vi "Actualizar Parametros.vi"(8 "error in (no error)":errorcluster, 10 "Parametros de la señal":T1, 11 "Generador de Señales in":refnum<class "Generador de Señales.lvclass">) -> (0 "error out":errorcluster, 3 "Generador de Señales out":refnum<class "Generador de Señales.lvclass">)   [LabVIEW 2020, in "Generador de Señales.lvlib" / "Generador de Señales.lvclass"]
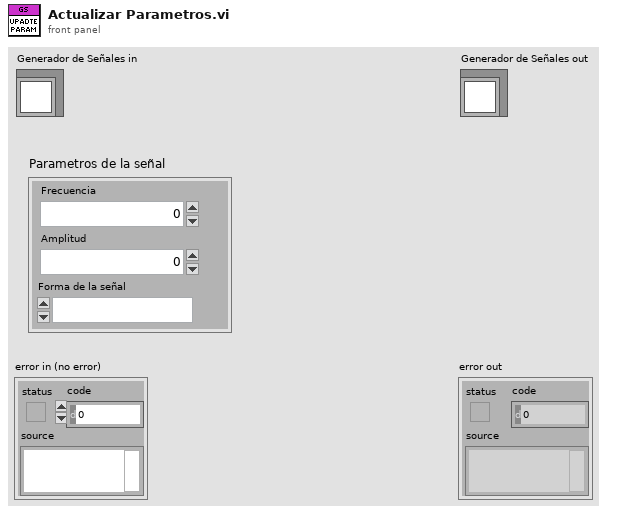
[diagram p1: front panel]
types:
  T1 = cluster{"Frecuencia":dbl, "Amplitud":dbl, "Forma de la señal":u16}
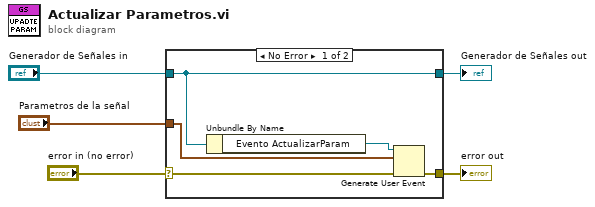
[diagram p0: block diagram]
diagram:
  n1 = case shown="No Error" "error in (no error)" {
    selector: "error in (no error)" -> [w9 w12]
    tunnel: [w8 w12] -> w4
    tunnel: [w10 w11] -> w2
    tunnel: "Generador de Señales in" -> [w10 w11]
    tunnel: "Parametros de la señal" -> [w6 _]
    frame No Error {
      n2 = Unbundle By Name(w10) -> ("Evento ActualizarParam"=w7:refnum<user-event>)
      n3 = Generate User Event(user event=w7, event data cluster=w6, error in=w9) -> (error out=w8:errorcluster)  [unwired: 1 in, 1 out]
    }
    frame Error {
    }
  }
  "error out" <- w4
  "Generador de Señales out" <- w2
